vi "Step.vi"(7 "input":T4, 9 "Nazwa":string, 10 "Numeric":i32) -> (1 "?":T1, 4 "output cluster":T3)   [LabVIEW 2020]
uses:
  controls/Data.ctl
panel:
  out "W cyklu":bool
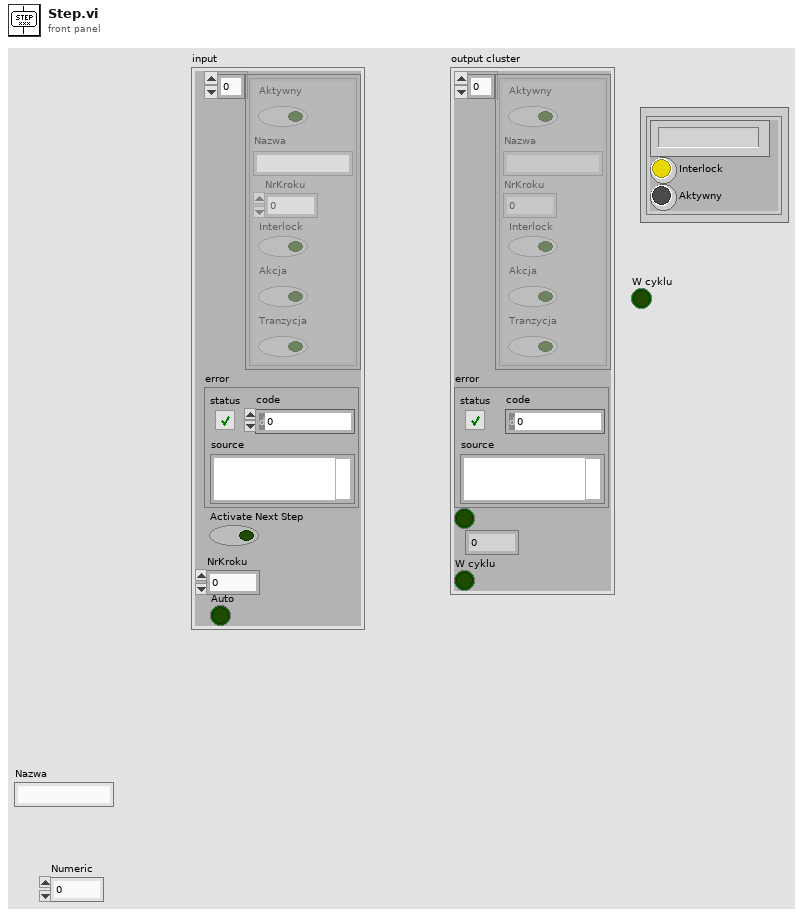
[diagram p1: front panel]
types:
  T1 = cluster{string, "Interlock":bool, "Aktywny":bool}
  T2 = typedef "Data.ctl" = cluster{"Aktywny":bool, "Nazwa":string, "NrKroku":dbl, "Interlock":bool, "Akcja":bool, "Tranzycja":bool}
  T3 = cluster{T2[], "error":errorcluster, bool, dbl, "W cyklu":bool}
  T4 = cluster{T2[], "error":errorcluster, "Activate Next Step":bool, "NrKroku":dbl, "Auto":bool}
  T5 = cluster{"Nazwa":string, "Interlock":bool, "Aktywny":bool}
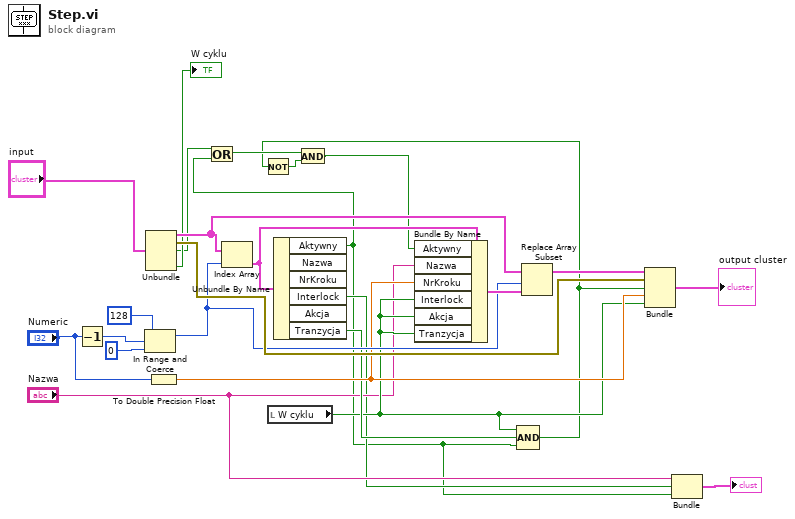
[diagram p0: block diagram]
diagram:
  n1 = Decrement(x="Numeric") -> (x-1=w16:i32)
  n2 = In Range and Coerce(upper limit=128, x=w16, lower limit=0) -> (coerced(x)=w21:i32)  [unwired: 1 out]
  n3 = Unbundle("input") -> (w20:T2[], "error"=w24:errorcluster, "Activate Next Step"=w9:bool, "Auto"=→"W cyklu":bool)  [unwired: 1 out]
  n4 = To Double Precision Float(number="Numeric") -> (double precision float=w15:dbl)
  n5 = Index Array(array=w20, index=w21) -> (element=w19:T2)
  n6 = local read "W cyklu"() -> (w13:bool)
  n7 = Unbundle By Name(w19) -> ("Aktywny"=w2:bool, "Interlock"=w3:bool, "Tranzycja"=w14:bool)  [unwired: 3 out]
  n8 = Or(x=w9, y=w2) -> (x .or. y?=w7:bool)
  n9 = Compound Arithmetic op=AND(w13, w14, w2) -> (w5:bool)
  n10 = Not(x=w5) -> (.not. x?=w6:bool)
  n11 = And(x=w7, y=w6) -> (x .and. y?=w8:bool)
  n12 = Bundle By Name(cluster=w19, "Aktywny"=w8, "Nazwa"="Nazwa", "NrKroku"=w15, "Interlock"=w13, "Akcja"=w13, "Tranzycja"=w13) -> (w22:T2)
  n13 = Replace Array Subset(array=w20, new element=w22, index=w21) -> (w23:T2[])
  n14 = Bundle(w23, "error"=w24, w5, w15, "W cyklu"=w13) -> (→"output cluster":T3)  [unwired: 1 in]
  n15 = Bundle("Nazwa"="Nazwa", "Interlock"=w3, "Aktywny"=w2) -> (→"?":T5)  [unwired: 1 in]
